vi "configuration UI.vi"() -> ()   [LabVIEW 2013, in "Scan Engine editor node.lvclass"]
uses:
  Scan Engine editor node.lvclass
  <vilib>/CEF_TreeControl/Node/NodeRef.ctl
  <vilib>/CEF_TreeControl/Node/NISE_CEF_Node.lvclass
  <vilib>/NI/AMC/Message Queue.ctl
  <vilib>/NI/AMC/Message.ctl
  <vilib>/NI/Tools/Keyed Array/KeyedArray.ctl
  <vilib>/CEF_TreeControl/Node/UserEventRef.ctl
  <vilib>/CEF_TreeControl/Controls/EventCluster.ctl
  <vilib>/NI/TBM Modules/variable/module/configuration/Scan Engine configuration.lvclass
  <vilib>/Utility/miscctls.llb/LVRowAndColumnUnsignedTypeDef.ctl
  <vilib>/NI/Module Execution Interface/Engine Configuration/engine configuration.lvclass
  <vilib>/NI/Tag Bus Data Framework/Configuration Editor/Classes/Engine Parent/Engine Parent Editor Node.lvclass
  <vilib>/NI/TBM Modules/variable/module/configuration/Scan Engine configuration.lvclass/Scan Engine configuration.ctl
  <vilib>/NI/Tag Bus Module Framework/root configuration/TBM configuration.lvclass/TBM configuration.ctl
  <vilib>/Utility/miscctls.llb/LVComboBoxStrsAndValuesArrayTypeDef.ctl
  <vilib>/NI/Tag Bus/tag/tag descriptor.lvclass/tag descriptor.ctl
  <vilib>/NI/Tag Bus/tag/write tag name.vi
  <vilib>/NI/TBM Modules/variable/module/configuration/Write discover channels.vi
  <vilib>/NI/TBM Modules/variable/module/configuration/Read discover channels.vi
  <vilib>/NI/Tag Bus Module Framework/root configuration/Read instance name.vi
  <vilib>/NI/Tag Bus Data Framework/Configuration Editor/Classes/Module editor node/Read Module Configuration.vi
  <vilib>/NI/Tag Bus Module Framework/root configuration/create GUID.vi
  <vilib>/NI/Tag Bus Data Framework/Configuration Editor/Classes/Module editor node/Write Module Configuration.vi
  <vilib>/NI/Tag Bus Data Framework/Configuration Editor/Classes/Engine Parent/write engine configuration.vi
  <vilib>/NI/Tag Bus Module Framework/root configuration/TBM configuration.lvclass
  <vilib>/NI/Tag Bus Module Framework/module configuration/TBM module configuration.lvclass
  <vilib>/NI/Tag Bus Data Framework/Configuration Editor/Classes/Module editor node/module editor node.lvclass
  <vilib>/NI/Tag Bus/tag/tag descriptor.lvclass
  <vilib>/CEF_TreeControl/NISE_CEF_TreeControl.lvlib
  <vilib>/NI/Tag Bus Module Framework/channel/TBM channel.lvclass
  <vilib>/NI/Tools/Keyed Array/Tools_KeyedArray.lvlib
  <vilib>/NI/AMC/AMC.lvlib
panel:
  in  "hidden_settings":bool
  in  "Tab Control":enum32{"Static Configuration"}(tab)
  in  "Generate Tags":bool
  in  "Discover Channels?":bool
  in  "Remove Button":bool
  in  "Add Button":bool
  in  "channels":i32(listbox)
  in  "settings":bool
  in  "Import":bool
  in  "Tag":string(combo)
  in  "scan period (uSec)":u32=10000
  in  "user event":T1
  in  "main queue":T2
  in  "node ref":T3
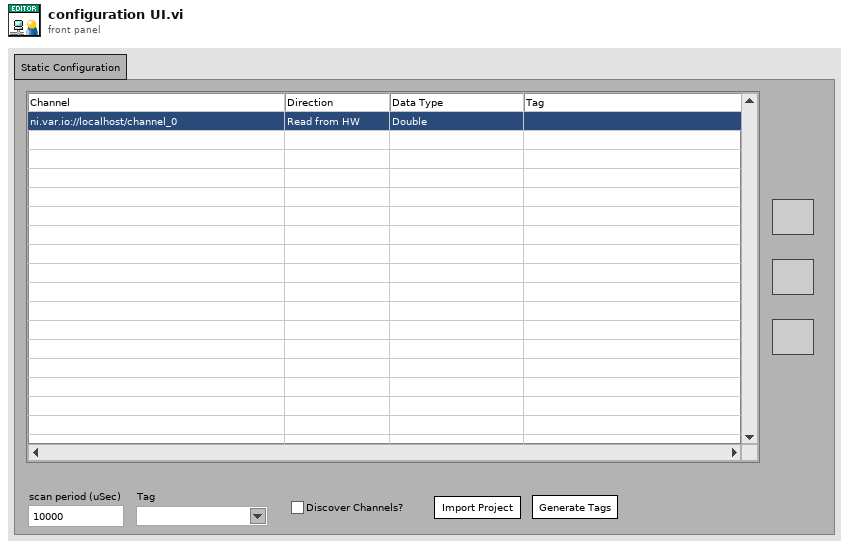
[diagram p1: front panel]
types:
  T1 = typedef "NISE_CEF_Node.lvclass/UserEventRef.ctl" = refnum<user-event>
  T2 = typedef "AMC.lvlib/Message Queue.ctl" = refnum<queue>
  T3 = typedef "NISE_CEF_Node.lvclass/NodeRef.ctl" = refnum<data-value>
  T4 = typedef "NISE_CEF_TreeControl.lvlib/EventCluster.ctl" = cluster{"command":string, "data":string}
  T5 = typedef "LVRowAndColumnUnsignedTypeDef.ctl" = cluster{"Row":u32, "Column":u32}
  T6 = typedef "LVComboBoxStrsAndValuesArrayTypeDef.ctl" = cluster{"String":string, "Value":string}[]
  T7 = typedef "Scan Engine editor node.lvclass/table line.ctl" = cluster{"tag":string, "channel":refnum<class "TBM channel.lvclass">}
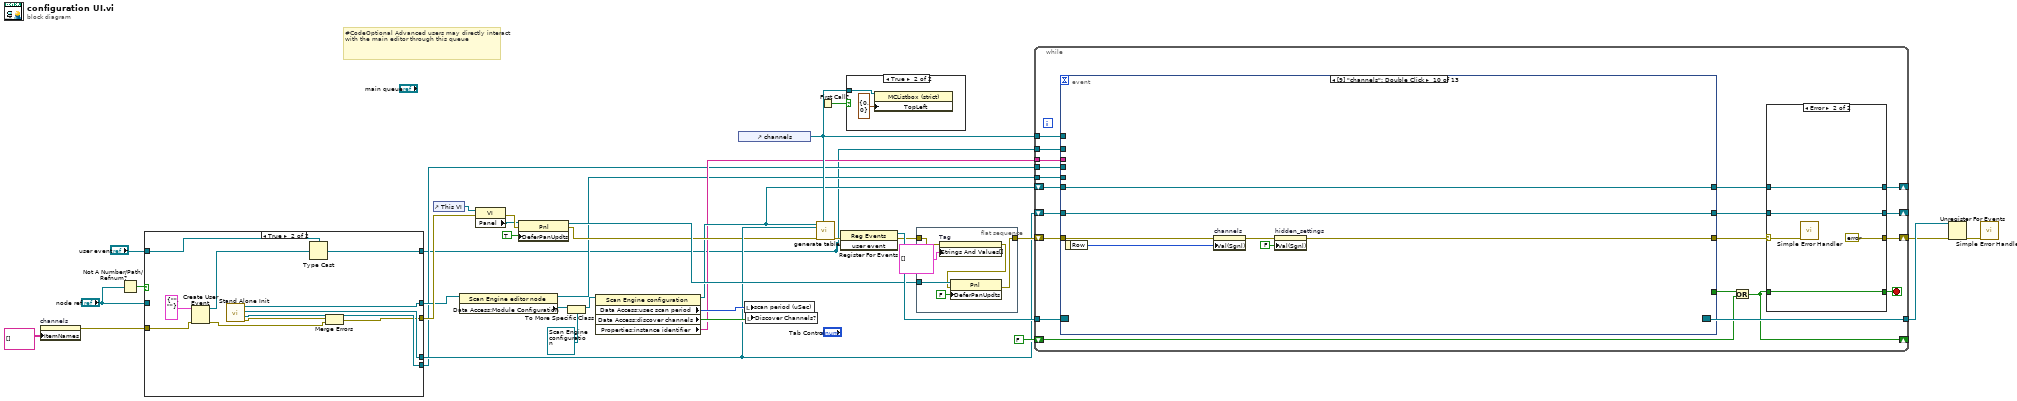
[diagram p0: block diagram]
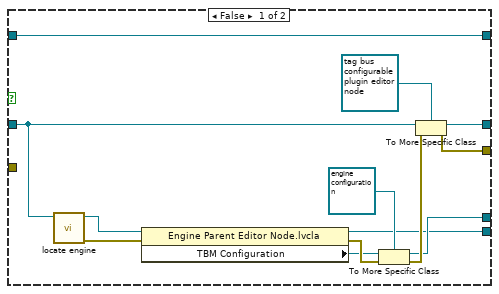
[diagram p2: hidden frame]
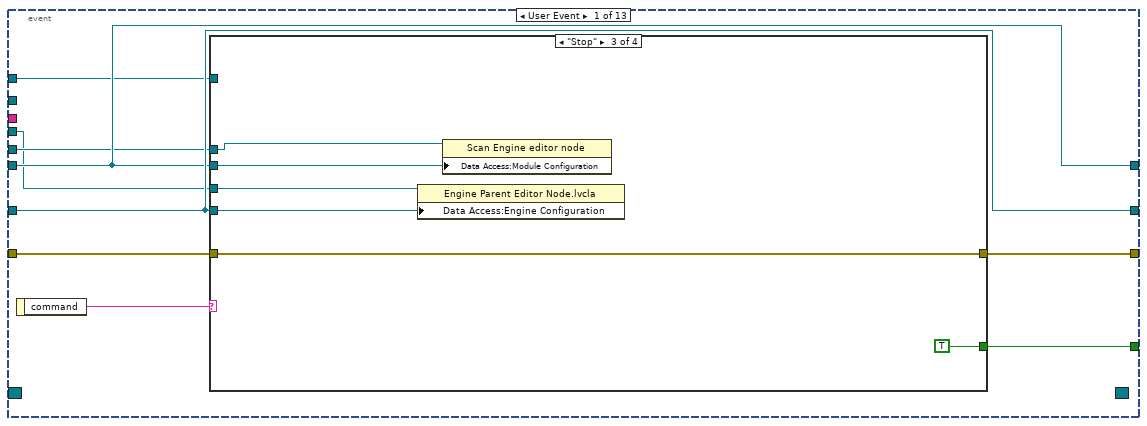
[diagram p5: hidden frame]
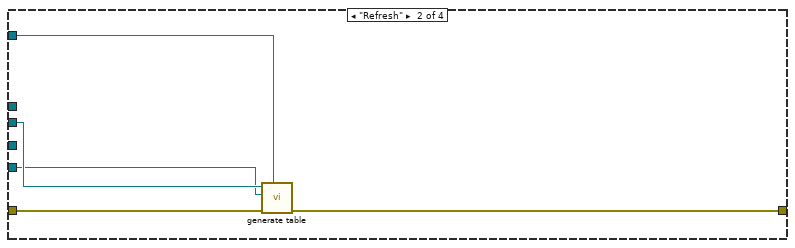
[diagram p7: hidden frame]
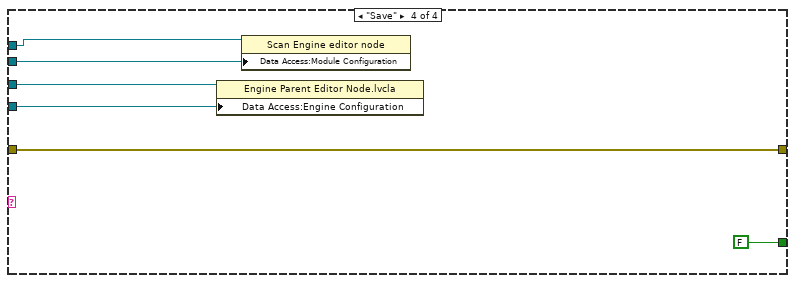
[diagram p8: hidden frame]
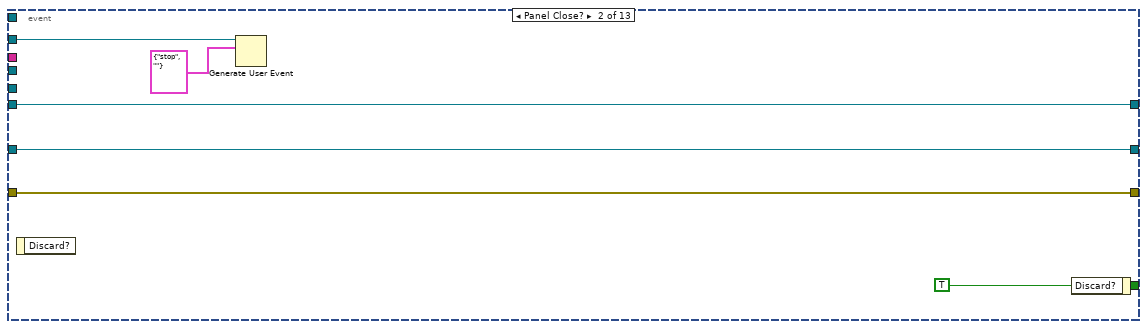
[diagram p9: hidden frame]
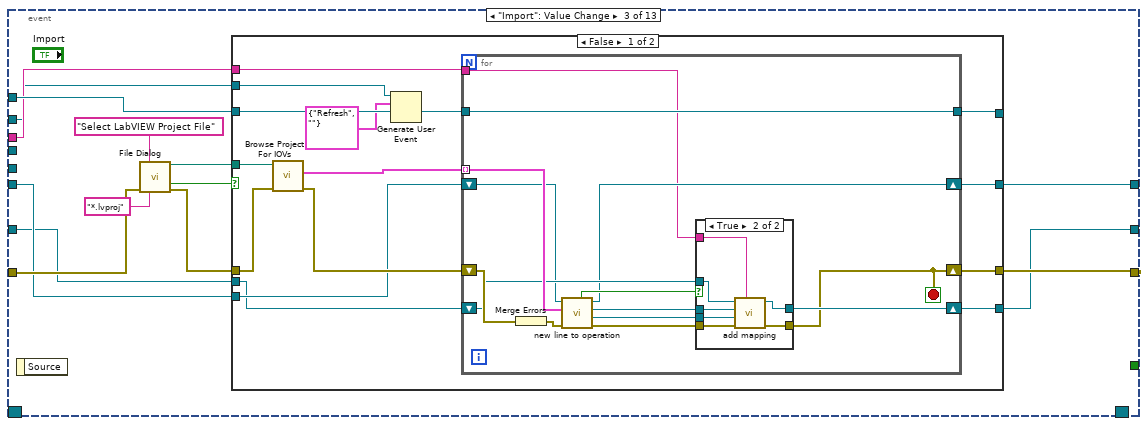
[diagram p10: hidden frame]
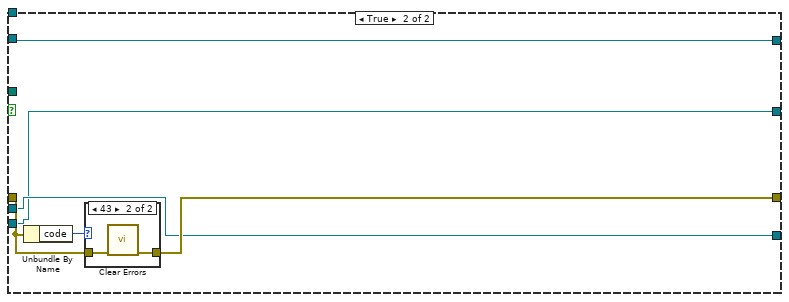
[diagram p12: hidden frame]
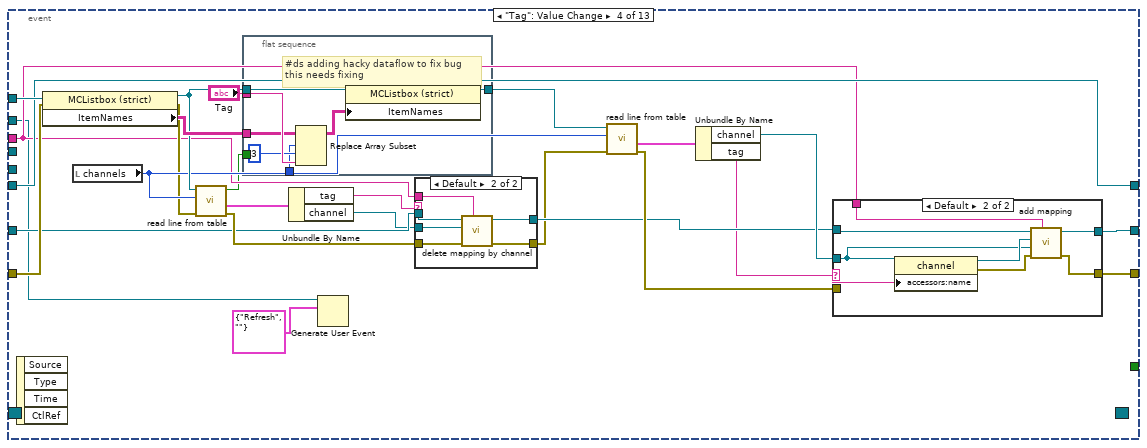
[diagram p14: hidden frame]
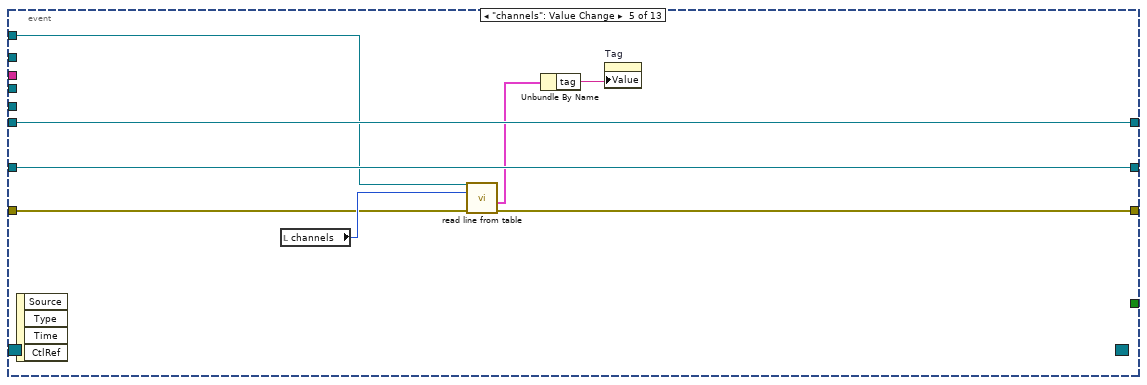
[diagram p17: hidden frame]
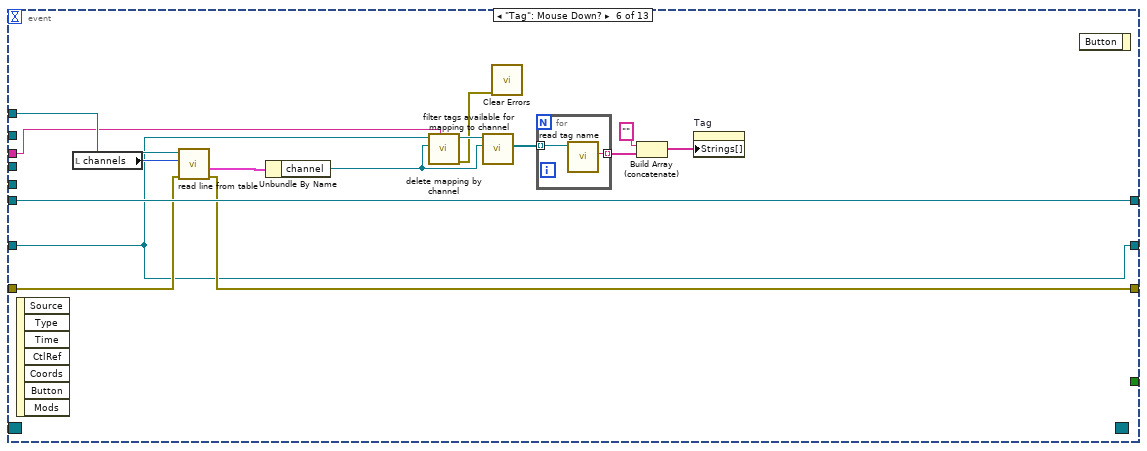
[diagram p18: hidden frame]
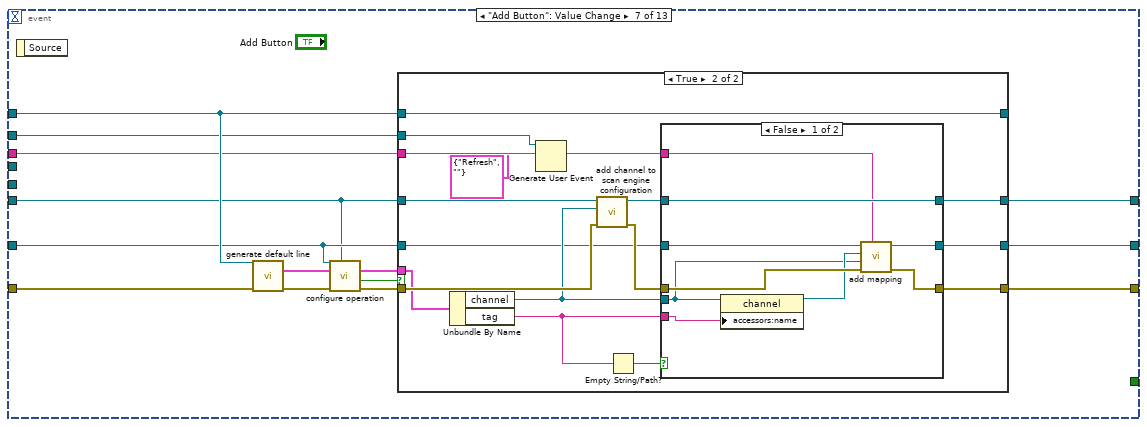
[diagram p19: hidden frame]
diagram:
  # "#CodeOptional Advanced users may directly interact with the main editor through this queue"
  n1 = property on="channels" class="MCListbox (strict)"("ItemNames"=string[][] [] ("Item Names")) -> (error out=w6:errorcluster)  [unwired: 2 in, 1 out]
  n2 = Not A Number/Path/Refnum?(number/path/refnum="node ref") -> (NaN/Path/Refnum?=w20:bool)
  n3 = case shown="True" w20 {
    tunnel: "user event" -> [w47 w48]
    tunnel: [w47 w49] -> w1
    tunnel: "node ref" -> [w45 _]
    tunnel: [w44 w58] -> w9
    tunnel: [w43 w51] -> w14
    tunnel: [w36 w56] -> w13
    tunnel: [w35 w55] -> w2
    tunnel: w6 -> [_ w52]
    frame False {
      n4 = call <vilib>:"locate engine.vi"("component"=w45) -> ("error out"=w40:errorcluster, "engine"=w42:refnum<data-value>)  [unwired: 9 in]
      n5 = property class="Engine Parent Editor Node.lvcla"(reference=w42, error in=w40) -> (reference out=w35:refnum<data-value>, error out=w39:errorcluster, "TBM Configuration"=w38:refnum<class "TBM configuration.lvclass">)
      n6 = To More Specific Class(target class=refnum<class "engine configuration.lvclass"> refnum ("engine configuration.lvclass"), reference=w38, error in=w39) -> (specific class reference=w36:refnum<class "engine configuration.lvclass">, error out=w37:errorcluster)
      n7 = To More Specific Class(target class=refnum<data-value> refnum ("data value reference"), reference=w45, error in=w37) -> (specific class reference=w44:refnum<data-value>, error out=w43:errorcluster)
    }
    frame True {
      n8 = Create User Event(user event datatype=T4 {"command"="", "data"=""} ("event data"), error in=w52) -> (user event=w53:refnum<user-event>, error out=w50:errorcluster)
      n9 = call "Stand Alone Init.vi"() -> ("error out"=w57:errorcluster, "Engine Parent Editor Node"=w55:refnum<data-value>, "engine configuration out"=w56:refnum<class "engine configuration.lvclass">, "Scan Engine Editor Node"=w58:refnum<data-value>)  [unwired: 8 in]
      n10 = Type Cast(type=w48, x=w53) -> (*(type *) &x=w49:T1)
      n11 = Merge Errors(w57, w50) -> (w51:errorcluster)
    }
  }
  n12 = control-ref of="This VI"() -> (w24:refnum<vi>)
  n13 = property class="Scan Engine editor node"(reference=w9) -> (reference out=w3:refnum<data-value>, "Data Access:Module Configuration"=w16:refnum<class "TBM module configuration.lvclass">)  [unwired: 1 in, 1 out]
  n14 = property class="VI"(reference=w24, error in=w14) -> (error out=w27:errorcluster, "Panel"=w26:refnum<vi>)  [unwired: 1 out]
  n15 = property class="Pnl"(reference=w26, error in=w27, "DeferPanUpdts"=TRUE ("Defer Panel Updates")) -> (reference out=w28:refnum<vi>, error out=w12:errorcluster)
  n16 = To More Specific Class(target class=refnum<class "Scan Engine configuration.lvclass"> refnum ("Scan Engine configuration"), reference=w16) -> (specific class reference=w15:refnum<class "Scan Engine configuration.lvclass">)  [unwired: 1 in, 1 out]
  n17 = property class="Scan Engine configuration"(reference=w15) -> (reference out=w8:refnum<class "Scan Engine configuration.lvclass">, "Data Access:usec scan period"=w22:u32, "Data Access:discover channels"=w21:bool, "Properties:instance identifier"=w7:string)  [unwired: 1 in, 1 out]
  n18 = control-ref of="channels"() -> (w10:refnum<vi>)
  n19 = local write "scan period (uSec)"(w22) -> ()
  n20 = local write "Discover Channels?"(w21) -> ()
  n21 = call "generate table.vi"("table"=w10, "error in"=w12, "engine configuration in"=w13, "Scan Engine configuration"=w8) -> ("error out"=w11:errorcluster)  [unwired: 7 in]
  n22 = First Call?() -> (First Call?: T/F=w23:bool)
  n23 = register-events(error in=w11, w1) -> (reference out=w34:refnum<event-registration>, error out=w30:errorcluster)  [unwired: 1 in]
  n24 = case shown="True" w23 {
    tunnel: w10 -> [_ w59]
    frame False {
    }
    frame True {
      n25 = property class="MCListbox (strict)"(reference=w59, "TopLeft"=T5 {"Row"=0, "Column"=0} ("Top Left Visible Cell")) -> ()  [unwired: 1 in, 2 out]
    }
  }
  n26 = flat-sequence {
    tunnel: w30 -> [w64]
    tunnel: [w61] -> w29
    tunnel: w28 -> [w65]
    frame #0 {
      n27 = property on="Tag" class="CmbBox"(error in=w64, "Strings And Values[]"=T6 [] ("Strings And Values []")) -> (error out=w62:errorcluster)  [unwired: 1 in, 1 out]
      n28 = property class="Pnl"(reference=w65, error in=w62, "DeferPanUpdts"=FALSE ("Defer Panel Updates")) -> (error out=w61:errorcluster)  [unwired: 1 out]
    }
  }
  n29 = while {
    tunnel: w34 -> [w86]
    tunnel: [w85] -> w33
    shift-right: [w79] -> w32
    shift-left: w29 -> [w84]
    shift-right: [w81] -> _
    shift-left: FALSE -> [w80]
    tunnel: w10 -> [w68]
    shift-right: [w74] -> _
    shift-left: w8 -> [w78]
    shift-right: [w76] -> _
    shift-left: w13 -> [w77]
    tunnel: w7 -> [w72]
    tunnel: w3 -> [w70]
    tunnel: w2 -> [w69]
    tunnel: w1 -> [w67]
    stop <- w83 stop-if-true
    n30 = event shown="[9] \"channels\": Double Click" {
      selector: w86 -> [_ _ _ _ _ _ _ _ _ _ _ _ _]
      dyn-events: [_ _ _ _ _ _ _ _ _ _ _ _ _] -> w85
      timeout: _ -> [_ _ _ _ _ _ _ _ _ _ _ _ _]
      tunnel: [w103 _ _ _ _ _ _ _ _ _ _ _ _] -> w82
      tunnel: [w100 w127 w138 w205 w245 w254 w278 w317 w362 w381 w390 w394 w398] -> w71
      tunnel: w84 -> [w101 w127 w142 w213 w246 w253 w277 w324 w366 w383 w389 w395 w407]
      tunnel: w68 -> [w96 _ w136 w214 w242 w258 w272 w312 w361 _ _ _ _]
      tunnel: w72 -> [_ _ w130 w192 _ w249 w268 w315 w357 _ _ _ w402]
      tunnel: w78 -> [w99 w126 w134 w197 w244 w262 w266 w321 w358 w384 w388 w396 w405]
      tunnel: w77 -> [w102 w128 w133 w200 w243 w251 w267 w320 w359 w385 w386 w393 w403]
      tunnel: [w99 w126 w131 w197 w244 w262 w269 w318 w363 w384 w387 w392 w404] -> w73
      tunnel: [w102 w128 w132 w199 w243 w251 w270 w319 w360 w385 w386 w393 w408] -> w75
      tunnel: w70 -> [w98 _ _ _ _ _ _ _ _ _ _ _ _]
      tunnel: w69 -> [w97 _ _ _ _ _ _ _ _ _ _ _ _]
      tunnel: w67 -> [_ w124 w129 w189 _ _ w265 w311 w355 _ _ _ w399]
      event User Event {
        n31 = event-data() -> ("command"=w104:string)  [unwired: 1 in]
        n32 = case shown="\"Stop\"" w104 {
          tunnel: [_ _ TRUE FALSE] -> w103
          tunnel: w102 -> [_ w108 w115 w121]
          tunnel: w101 -> [w105 w107 w114 w120]
          tunnel: [w105 w106 w114 w120] -> w100
          tunnel: w99 -> [_ w109 w113 w119]
          tunnel: w98 -> [_ _ w111 w117]
          tunnel: w97 -> [_ _ w112 w118]
          tunnel: w96 -> [_ w110 _ _]
          frame Default {
          }
          frame "Refresh" {
            n33 = call "generate table.vi"("table"=w110, "error in"=w107, "engine configuration in"=w108, "Scan Engine configuration"=w109) -> ("error out"=w106:errorcluster)  [unwired: 7 in]
          }
          frame "Stop" {
            n34 = property class="Engine Parent Editor Node.lvcla"(reference=w112, "Data Access:Engine Configuration"=w115) -> ()  [unwired: 1 in, 2 out]
            n35 = property class="Scan Engine editor node"(reference=w111, "Data Access:Module Configuration"=w113) -> ()  [unwired: 1 in, 2 out]
          }
          frame "Save" {
            n36 = property class="Engine Parent Editor Node.lvcla"(reference=w118, "Data Access:Engine Configuration"=w121) -> ()  [unwired: 1 in, 2 out]
            n37 = property class="Scan Engine editor node"(reference=w117, "Data Access:Module Configuration"=w119) -> ()  [unwired: 1 in, 2 out]
          }
        }
      }
      event Panel Close? {
        n38 = event-data() -> ()  [unwired: 1 in, 1 out]
        n39 = Generate User Event(user event=w124, event data cluster=T4 {"command"="stop", "data"=""} ("event data")) -> ()  [unwired: 2 in, 2 out]
        n40 = event-data("Discard?"=TRUE) -> ()  [unwired: 1 in, 1 out]
      }
      event "Import": Value Change {
        n41 = event-data() -> ()  [unwired: 1 in, 1 out]
        n42 = call "File Dialog"("prompt"="Select LabVIEW Project File", "error in"=w142, "pattern (all files)"="*.lvproj") -> ("selected path"=w137:path, "cancelled"=w140:bool, "error out"=w139:errorcluster)  [unwired: 9 in, 1 out]
        n43 = case shown="False" w140 {
          tunnel: w139 -> [w155 w184]
          tunnel: [w151 w183] -> w138
          tunnel: w137 -> [w156 _]
          tunnel: w136 -> [w153 w180]
          tunnel: w130 -> [w150 _]
          tunnel: w134 -> [w149 w181]
          tunnel: w133 -> [w148 w182]
          tunnel: [w147 w182] -> w132
          tunnel: [w146 w180] -> _
          tunnel: [w145 w181] -> w131
          tunnel: w129 -> [w143 _]
          frame False {
            n44 = call "Browse Project For IOVs.vi"("error in"=w155, "Path"=w156) -> ("error out"=w154:errorcluster, "Tags"=w152:T7[])  [unwired: 8 in]
            n45 = Generate User Event(user event=w143, event data cluster=T4 {"command"="Refresh", "data"=""} ("event data")) -> ()  [unwired: 2 in, 2 out]
            n46 = for {
              tunnel: w152 -> [w166] mode=indexing
              shift-right: [w160] -> w151
              shift-left: w154 -> [w169]
              tunnel: w153 -> [w161]
              tunnel: w150 -> [w157]
              tunnel: [w161] -> w146
              shift-right: [w164] -> w147
              shift-left: w148 -> [w165]
              shift-right: [w158] -> w145
              shift-left: w149 -> [w159]
              stop <- w160 stop-if-true
              n47 = Merge Errors(w169) -> (w168:errorcluster)
              n48 = call "new line to operation.vi"("error in"=w168, "new line item"=w166, "Actual Configuration"=w159) -> ("error out"=w170:errorcluster, "channel"=w162:refnum<class "TBM channel.lvclass">, "Tag reference"=w163:refnum<class "tag descriptor.lvclass">, "Scan Engine configuration out"=w158:refnum<class "Scan Engine configuration.lvclass">, "new mapping?"=w167:bool)  [unwired: 4 in]
              n49 = case shown="True" w167 {
                tunnel: w170 -> [w172 w178]
                tunnel: [w172 w179] -> w160
                tunnel: w165 -> [w171 w177]
                tunnel: [w171 w176] -> w164
                tunnel: w163 -> [_ w175]
                tunnel: w162 -> [_ w174]
                tunnel: w157 -> [_ w173]
                frame False {
                }
                frame True {
                  n50 = call <vilib>:"add mapping.vi"("owner ID"=w173, "error in"=w178, "channel"=w174, "tag descriptor"=w175, "engine configuration"=w177) -> ("error out"=w179:errorcluster, "engine configuration out"=w176:refnum<class "engine configuration.lvclass">)  [unwired: 5 in]
                }
              }
            }
          }
          frame True {
            n51 = Unbundle By Name(w184) -> ("code"=w185:i32)
            n52 = case shown="43" w185 {
              tunnel: w184 -> [w186 w188]
              tunnel: [w186 w187] -> w183
              frame Default {
              }
              frame 43 {
                n53 = call <vilib>:"Clear Errors.vi"("error in (no error)"=w188) -> ("error out"=w187:errorcluster)  [unwired: 6 in]
              }
            }
          }
        }
      }
      event "Tag": Value Change {
        n54 = event-data() -> ()  [unwired: 1 in, 4 out]
        n55 = property class="MCListbox (strict)"(reference=w214, error in=w213) -> (reference out=w210:refnum<vi>, error out=w208:errorcluster, "ItemNames"=w211:string[][])
        n56 = local read "channels"() -> (w209:i32)
        n57 = call "read line from table.vi"("error in"=w208, "line number"=w209, "operations table"=w210) -> ("error out"=w207:errorcluster, "line"=w204:T7, "empty channel?"=w191:bool)  [unwired: 5 in, 1 out]
        n58 = flat-sequence {
          tunnel: "Tag" -> [w221]
          tunnel: w211 -> [w219]
          tunnel: w210 -> [w217]
          tunnel: w209 -> [w216]
          tunnel: [w215] -> w196
          tunnel: w191 -> [_]
          frame #0 {
            # "#ds adding hacky dataflow to fix bug\nthis needs fixing"
            n59 = Replace Array Subset(array=w219, new element=w221, index (row)=w216, index (col)=3 ("disabled index (col)")) -> (w220:string[][])
            n60 = property class="MCListbox (strict)"(reference=w217, "ItemNames"=w220) -> (reference out=w215:refnum<vi>)  [unwired: 1 in, 1 out]
          }
        }
        n61 = Unbundle By Name(w204) -> ("tag"=w195:string, "channel"=w194:refnum<class "TBM channel.lvclass">)
        n62 = Generate User Event(user event=w189, event data cluster=T4 {"command"="Refresh", "data"=""} ("event data")) -> ()  [unwired: 2 in, 2 out]
        n63 = case shown="Default" w195 {
          tunnel: [w233 w234] -> w193
          tunnel: w192 -> [_ w235]
          tunnel: w207 -> [w233 w239]
          tunnel: [w232 w238] -> w201
          tunnel: w200 -> [w232 w237]
          tunnel: w194 -> [_ w236]
          frame "" {
          }
          frame Default {
            n64 = call <vilib>:"delete mapping by channel.vi"("owner ID"=w235, "error in"=w239, "channel"=w236, "engine configuration in"=w237) -> ("error out"=w234:errorcluster, "engine configuration out"=w238:refnum<class "engine configuration.lvclass">)  [unwired: 6 in]
          }
        }
        n65 = call "read line from table.vi"("error in"=w193, "line number"=w209, "operations table"=w196) -> ("error out"=w206:errorcluster, "line"=w203:T7)  [unwired: 5 in, 2 out]
        n66 = Unbundle By Name(w203) -> ("channel"=w202:refnum<class "TBM channel.lvclass">, "tag"=w198:string)
        n67 = case shown="Default" w198 {
          selector: w198 -> [_ w226]
          tunnel: [w223 w227] -> w205
          tunnel: w206 -> [w223 _]
          tunnel: w202 -> [_ w230]
          tunnel: w201 -> [w222 w228]
          tunnel: [w222 w229] -> w199
          tunnel: w192 -> [_ w224]
          frame "" {
          }
          frame Default {
            n68 = property class="channel"(reference=w230, "accessors:name"=w226) -> (reference out=w231:refnum<class "TBM channel.lvclass">, error out=w225:errorcluster)  [unwired: 1 in]
            n69 = call <vilib>:"add mapping.vi"("owner ID"=w224, "error in"=w225, "channel"=w230, "tag descriptor"=w231, "engine configuration"=w228) -> ("error out"=w227:errorcluster, "engine configuration out"=w229:refnum<class "engine configuration.lvclass">)  [unwired: 5 in]
          }
        }
      }
      event "channels": Value Change {
        n70 = event-data() -> ()  [unwired: 1 in, 4 out]
        n71 = local read "channels"() -> (w247:i32)
        n72 = call "read line from table.vi"("error in"=w246, "line number"=w247, "operations table"=w242) -> ("error out"=w245:errorcluster, "line"=w241:T7)  [unwired: 5 in, 2 out]
        n73 = Unbundle By Name(w241) -> ("tag"=w240:string)
        n74 = property on="Tag" class="CmbBox"("Value"=w240) -> ()  [unwired: 2 in, 2 out]
      }
      event "Tag": Mouse Down? {
        n75 = event-data() -> ()  [unwired: 1 in, 7 out]
        n76 = local read "channels"() -> (w257:i32)
        n77 = call "read line from table.vi"("error in"=w253, "line number"=w257, "operations table"=w258) -> ("error out"=w254:errorcluster, "line"=w256:T7)  [unwired: 5 in, 2 out]
        n78 = Unbundle By Name(w256) -> ("channel"=w250:refnum<class "TBM channel.lvclass">)
        n79 = call <vilib>:"delete mapping by channel.vi"("owner ID"=w249, "channel"=w250, "engine configuration in"=w251) -> ("error out"=w248:errorcluster, "engine configuration out"=w252:refnum<class "engine configuration.lvclass">)  [unwired: 7 in]
        n80 = call <vilib>:"filter tags available for mapping to channel.vi"("channel to map to"=w250, "engine configuration in"=w252) -> ("filtered tags"=w261:refnum<class "tag descriptor.lvclass">[])  [unwired: 8 in, 1 out]
        n81 = call <vilib>:"Clear Errors.vi"("error in (no error)"=w248) -> ()  [unwired: 6 in, 1 out]
        n82 = for {
          tunnel: w261 -> [w264] mode=indexing
          tunnel: [w263] -> w260 mode=indexing
          n83 = call <vilib>:"read tag name.vi"("system tag in"=w264) -> ("name"=w263:string)  [unwired: 8 in, 2 out]
        }
        n84 = Build Array (concatenate)("", w260) -> (w255:string[])
        n85 = property on="Tag" class="CmbBox"("Strings[]"=w255) -> ()  [unwired: 2 in, 2 out]
        n86 = event-data() -> ()  [unwired: 2 in, 1 out]
      }
      event "Add Button": Value Change {
        n87 = event-data() -> ()  [unwired: 1 in, 1 out]
        n88 = call "generate default line.vi"("error in"=w277, "operations table"=w272) -> ("error out"=w275:errorcluster, "line item in"=w271:T7)  [unwired: 8 in]
        n89 = call "configure operation.vi"("Scan Engine configuration"=w266, "error in"=w275, "line item in"=w271, "engine configuration in"=w267) -> ("error out"=w276:errorcluster, "success"=w274:bool, "line item out"=w273:T7)  [unwired: 4 in, 1 out]
        n90 = case shown="True" w274 {
          tunnel: [w282 w288] -> w278
          tunnel: [w281 w286] -> w269
          tunnel: w272 -> [w279 w287]
          tunnel: w276 -> [w282 w295]
          tunnel: w267 -> [w280 w292]
          tunnel: w273 -> [_ w294]
          tunnel: w268 -> [_ w298]
          tunnel: w266 -> [w281 w297]
          tunnel: [w280 w289] -> w270
          tunnel: [w279 w287] -> _
          tunnel: w265 -> [_ w283]
          frame False {
          }
          frame True {
            n91 = Unbundle By Name(w294) -> ("channel"=w293:refnum<class "TBM channel.lvclass">, "tag"=w291:string)
            n92 = Generate User Event(user event=w283, event data cluster=T4 {"command"="Refresh", "data"=""} ("event data")) -> ()  [unwired: 2 in, 2 out]
            n93 = call <vilib>:"add channel to scan engine configuration.vi"("error in"=w295, "channel"=w293, "Scan Engine configuration in"=w297) -> ("error out"=w296:errorcluster, "Scan Engine configuration out"=w285:refnum<class "Scan Engine configuration.lvclass">)  [unwired: 7 in]
            n94 = Empty String/Path?(string/path=w291) -> (empty?=w290:bool)
            n95 = case shown="False" w290 {
              tunnel: w296 -> [w307 w310]
              tunnel: [w306 w310] -> w288
              tunnel: w298 -> [w299 _]
              tunnel: w293 -> [w302 _]
              tunnel: w291 -> [w305 _]
              tunnel: w292 -> [w303 w309]
              tunnel: [w301 w309] -> w289
              tunnel: [w300 w308] -> w286
              tunnel: w285 -> [w300 w308]
              frame False {
                n96 = property class="channel"(reference=w302, "accessors:name"=w305) -> (reference out=w304:refnum<class "TBM channel.lvclass">)  [unwired: 1 in, 1 out]
                n97 = call <vilib>:"add mapping.vi"("owner ID"=w299, "error in"=w307, "channel"=w302, "tag descriptor"=w304, "engine configuration"=w303) -> ("error out"=w306:errorcluster, "engine configuration out"=w301:refnum<class "engine configuration.lvclass">)  [unwired: 5 in]
              }
              frame True {
              }
            }
          }
        }
      }
      event "Remove Button": Value Change {
        n98 = event-data() -> ()  [unwired: 1 in, 1 out]
        n99 = local read "channels"() -> (w323:i32)
        n100 = call "read line from table.vi"("error in"=w324, "line number"=w323, "operations table"=w312) -> ("error out"=w322:errorcluster, "line"=w316:T7, "empty tag?"=w313:bool, "empty channel?"=w314:bool)  [unwired: 5 in]
        n101 = case shown="False" w314 {
          tunnel: w322 -> [w338 w351]
          tunnel: w321 -> [w337 w353]
          tunnel: w320 -> [w336 w352]
          tunnel: [w335 w352] -> w319
          tunnel: [w330 w353] -> w318
          tunnel: [w334 w351] -> w317
          tunnel: w316 -> [w333 _]
          tunnel: w315 -> [w332 _]
          tunnel: w313 -> [w328 _]
          tunnel: [w327 w350] -> _
          tunnel: w312 -> [w327 w350]
          tunnel: w311 -> [w325 _]
          frame False {
            n102 = Generate User Event(user event=w325, event data cluster=T4 {"command"="Refresh", "data"=""} ("event data")) -> ()  [unwired: 2 in, 2 out]
            n103 = Unbundle By Name(w333) -> ("channel"=w331:refnum<class "TBM channel.lvclass">)
            n104 = call <vilib>:"delete channel from configuration.vi"("error in"=w338, "channel"=w331, "Scan Engine configuration in"=w337) -> ("error out"=w339:errorcluster, "Scan Engine configuration out"=w329:refnum<class "Scan Engine configuration.lvclass">)  [unwired: 7 in]
            n105 = case shown="False" w328 {
              tunnel: w339 -> [w346 w347]
              tunnel: w336 -> [w345 w349]
              tunnel: [w344 w349] -> w335
              tunnel: [w343 w347] -> w334
              tunnel: w332 -> [w340 _]
              tunnel: w331 -> [w342 _]
              tunnel: [w341 w348] -> w330
              tunnel: w329 -> [w341 w348]
              frame False {
                n106 = call <vilib>:"delete mapping by channel.vi"("owner ID"=w340, "error in"=w346, "channel"=w342, "engine configuration in"=w345) -> ("error out"=w343:errorcluster, "engine configuration out"=w344:refnum<class "engine configuration.lvclass">)  [unwired: 6 in]
              }
              frame True {
              }
            }
          }
          frame True {
          }
        }
      }
      event "settings", "hidden_settings": Value Change {
        n107 = event-data() -> ()  [unwired: 1 in, 1 out]
        n108 = call "read line from table.vi"("error in"=w366, "line number"="channels", "operations table"=w361) -> ("error out"=w365:errorcluster, "line"=w356:T7, "empty channel?"=w354:bool)  [unwired: 5 in, 1 out]
        n109 = case shown="True" w354 {
          tunnel: w365 -> [w375 w376]
          tunnel: [w374 w378] -> w363
          tunnel: [w373 w376] -> w362
          tunnel: [w372 w377] -> w360
          tunnel: w359 -> [w371 w377]
          tunnel: w358 -> [w370 w378]
          tunnel: w357 -> [w369 _]
          tunnel: w356 -> [w368 _]
          tunnel: w355 -> [w367 _]
          frame False {
            n110 = call "configure channel.vi"("user event"=w367, "instance id"=w369, "error in"=w375, "line"=w368, "engine configuration in"=w371, "Scan Engine configuration in"=w370) -> ("error out"=w373:errorcluster, "engine configuration out"=w372:refnum<class "engine configuration.lvclass">, "Scan Engine configuration out"=w374:refnum<class "Scan Engine configuration.lvclass">)  [unwired: 3 in]
          }
          frame True {
          }
        }
      }
      event "channels": Double Click {
        n111 = event-data() -> ("Row"=w379:i32)  [unwired: 1 in]
        n112 = property on="channels" class="MCListbox (strict)"(error in=w383, "Val(Sgnl)"=w379) -> (error out=w382:errorcluster)  [unwired: 1 in, 1 out]
        n113 = property on="hidden_settings" class="Bool (strict)"(error in=w382, "Val(Sgnl)"=FALSE ("Value (Signaling)")) -> (error out=w381:errorcluster)  [unwired: 1 in, 1 out]
      }
      event "scan period (uSec)": Value Change {
        n114 = event-data() -> ()  [unwired: 1 in, 1 out]
        n115 = property class="Scan Engine configuration"(reference=w388, error in=w389, "Data Access:usec scan period"="scan period (uSec)") -> (reference out=w387:refnum<class "Scan Engine configuration.lvclass">, error out=w390:errorcluster)
      }
      event "Discover Channels?": Value Change {
        n116 = event-data() -> ()  [unwired: 1 in, 3 out]
        n117 = property class="Scan Engine configuration"(reference=w396, error in=w395, "Data Access:discover channels"="Discover Channels?") -> (reference out=w392:refnum<class "Scan Engine configuration.lvclass">, error out=w394:errorcluster)
      }
      event "Generate Tags": Value Change {
        # "#todo Create an engine filter VI that returns all channels that are currently mapped."
        n118 = event-data() -> ()  [unwired: 1 in, 1 out]
        n119 = call-dynamic "get channels.vi"("module configuration in"=w405) -> ("channels"=w401:refnum<class "TBM channel.lvclass">[], "module configuration out"=w404:refnum<class "Scan Engine configuration.lvclass">)  [unwired: 9 in]
        n120 = Generate User Event(user event=w399, event data cluster=T4 {"command"="Refresh", "data"=""} ("event data")) -> ()  [unwired: 2 in, 2 out]
        n121 = for {
          tunnel: w401 -> [w412] mode=indexing
          shift-right: [w416] -> w408
          shift-left: w403 -> [w414]
          tunnel: w402 -> [w413]
          tunnel: w407 -> [w409]
          tunnel: [w415] -> w406 mode=indexing
          n122 = call <vilib>:"find tag mapped to channel.vi"("owner"=w413, "error in"=w409, "channel"=w412, "engine configuration in"=w414) -> ("error out"=w410:errorcluster, "engine configuration out"=w411:refnum<class "engine configuration.lvclass">)  [unwired: 5 in, 1 out]
          n123 = case shown="No Error" w410 {
            selector: w410 -> [w417 _]
            tunnel: [w418 w424] -> w416
            tunnel: [w417 w423] -> w415
            tunnel: w413 -> [_ w422]
            tunnel: w412 -> [_ w421]
            tunnel: w411 -> [w418 w420]
            tunnel: w409 -> [_ w419]
            frame No Error {
            }
            frame Error {
              n124 = call <vilib>:"add tag.vi"("error in"=w419, "tag descriptor"=w421, "engine configuration in"=w420) -> ("error out"=w425:errorcluster, "engine configuration out"=w426:refnum<class "engine configuration.lvclass">)  [unwired: 7 in]
              n125 = call <vilib>:"add mapping.vi"("owner ID"=w422, "error in"=w425, "channel"=w421, "tag descriptor"=w421, "engine configuration"=w426) -> ("error out"=w423:errorcluster, "engine configuration out"=w424:refnum<class "engine configuration.lvclass">)  [unwired: 5 in]
            }
          }
        }
        n126 = Merge Errors(w406) -> (w398:errorcluster)
      }
    }
    n127 = Or(x=w82, y=w80) -> (x .or. y?=w81:bool)
    n128 = case shown="Error" w71 {
      selector: w71 -> [w89 w94]
      tunnel: [w90 w95] -> w83
      tunnel: w81 -> [w90 w95]
      tunnel: [w89 errorcluster {"status"=FALSE, "code"=0, "source"=""} ("error out")] -> w79
      tunnel: [w88 w91] -> w76
      tunnel: w75 -> [w88 w91]
      tunnel: [w87 w92] -> w74
      tunnel: w73 -> [w87 w92]
      frame No Error {
      }
      frame Error {
        n129 = call <vilib>:"Simple Error Handler.vi"("error in (no error)"=w94) -> ()  [unwired: 4 in, 5 out]
      }
    }
  }
  n130 = Unregister For Events(event registration refnum=w33, error in=w32) -> (error out=w4:errorcluster)
  n131 = call <vilib>:"Simple Error Handler.vi"("error in (no error)"=w4) -> ()  [unwired: 4 in, 5 out]
